vi "GV_PlotRscale.vi"(8 "error in (no error)":errorcluster, 11 "Gviewer in":refnum<class "Gviewer.lvclass">) -> (0 "error out":errorcluster, 3 "Gviewer out":refnum<class "Gviewer.lvclass">)   [LabVIEW 2020, in "Sgraph_lib_V1.lvlib" / "Gviewer.lvclass"]
doc: "Andre Koelewijn, 17 feb 2022,\n\nPlot Right Scale data if selected"
uses:
  Gviewer.lvclass
  Gviewer.lvclass/Gviewer.ctl
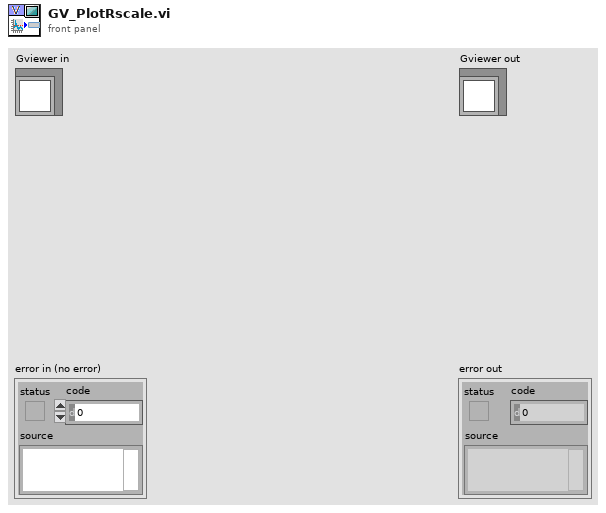
[diagram p1: front panel]
types:
  T1 = typedef "Sgraph_lib_V1.lvlib/Gviewer.lvclass/TD_Rscale.ctl" = enum16{"none", "one", "all"}
  T2 = typedef "Sgraph_lib_V1.lvlib/Gviewer.lvclass/Typedef_SelProperties.ctl" = cluster{"Color":u32, "LineType":T3, "max":dbl, "min":dbl, "unit":string}
  T3 = typedef "Sgraph_lib_V1.lvlib/Gviewer.lvclass/Typedef_LineType.ctl" = enum16{"num_bare", "num_MinMax_Area", "num_MinMax_Lines", "num_MinMax_Forfor", "num_Max_Area", "num_Max_Line", "num_Max_Forfor", "num_Min_Area", "num_Min_Line", "num_Min_Fosfor", "Boolean_Line_01", "Boolean_Area_01", "Boolean_Fosfor_01", "Boolean_Line_TF", "Boolean_Area_TF", "Boolean_Fosfor_TF", "Boolean_OnOff_Line", "Boolean_OnOff_Area", "Boolean_OnOff_Fosfor", "Boolean_spare", "StringEvent_Line", "StringEvent_TimeLine"}
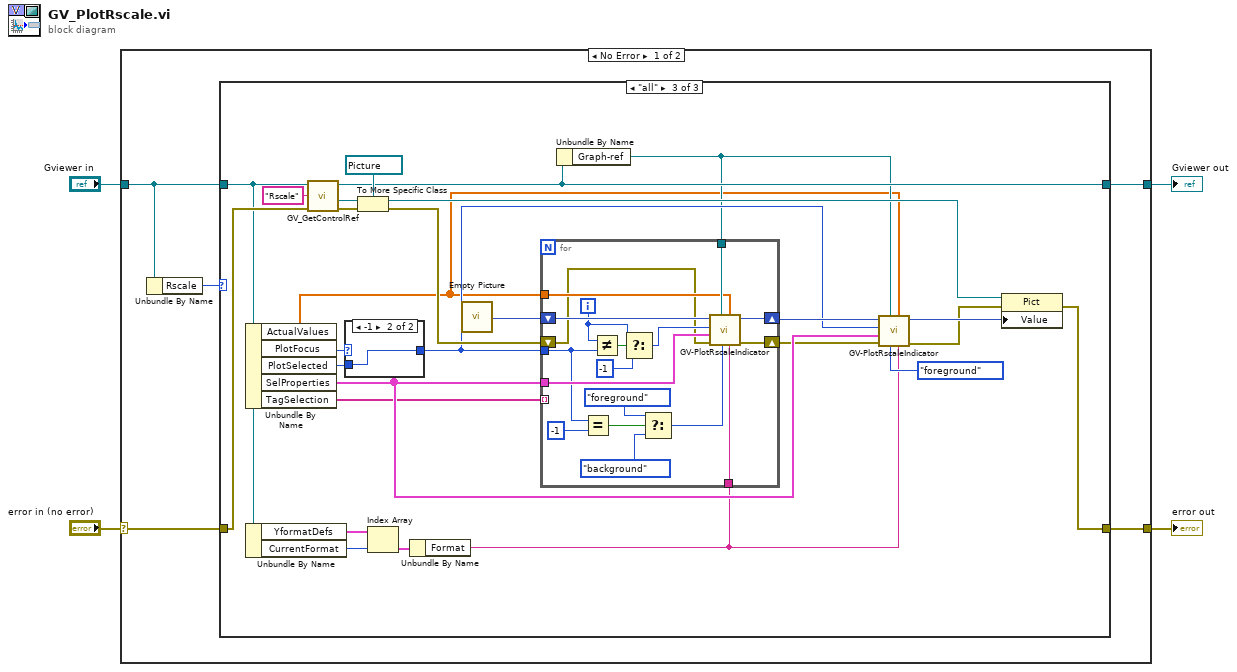
[diagram p0: block diagram]
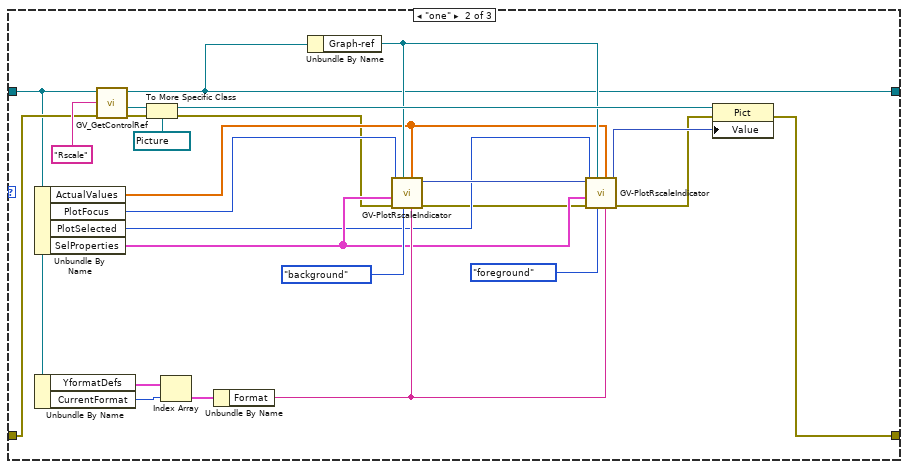
[diagram p3: hidden frame]
diagram:
  n1 = case shown="No Error" "error in (no error)" {
    selector: "error in (no error)" -> [w6 w85]
    tunnel: [w5 w85] -> w3
    tunnel: [w7 w84] -> w1
    tunnel: "Gviewer in" -> [w8 w84]
    frame No Error {
      n2 = Unbundle By Name(w8) -> ("Rscale"=w9:T1)
      n3 = case shown="\"all\"" w9 {
        tunnel: w8 -> [w11 w24 w55]
        tunnel: [w11 w12 w57] -> w7
        tunnel: w6 -> [w10 w31 w58]
        tunnel: [w10 w36 w63] -> w5
        frame Default {
        }
        frame "one" {
          n4 = Unbundle By Name(w24) -> ("ActualValues"=w17:dbl[], "PlotFocus"=w16:i32, "PlotSelected"=w15:i32, "SelProperties"=w18:T2[])
          n5 = Unbundle By Name(w24) -> ("YformatDefs"=w27:cluster{"Description":string, "Format":string}[], "CurrentFormat"=w26:i32)
          n6 = call "GV_GetControlRef.vi"("error in (no error)"=w31, "CNT name"="Rscale", "Gviewer in"=w24) -> ("error out"=w35:errorcluster, "Reference"=w34:refnum<vi>, "Gviewer out"=w12:refnum<class "Gviewer.lvclass">)  [unwired: 6 in]
          n7 = To More Specific Class(target class=refnum<vi> refnum ("2D Picture"), reference=w34, error in=w35) -> (specific class reference=w28:refnum<vi>, error out=w14:errorcluster)
          n8 = Index Array(array=w27, index=w26) -> (element=w25:cluster{"Description":string, "Format":string})
          n9 = Unbundle By Name(w25) -> ("Format"=w20:string)
          n10 = Unbundle By Name(w12) -> ("Graph-ref"=w21:refnum<vi>)
          n11 = call "GV-PlotRscaleIndicator.vi"("Format"=w20, "ActualValues"=w17, "type"=enum16{"background", "foreground"}."background", "Graph-ref"=w21, "error in (no error)"=w14, "SelProperties"=w18, "Plot"=w16) -> ("error out"=w13:errorcluster, "Picture OUT"=w23:picture)  [unwired: 3 in]
          n12 = call "GV-PlotRscaleIndicator.vi"("Format"=w20, "ActualValues"=w17, "type"=enum16{"background", "foreground"}."foreground", "Graph-ref"=w21, "error in (no error)"=w13, "SelProperties"=w18, "Plot"=w15, "Picture IN"=w23) -> ("error out"=w29:errorcluster, "Picture OUT"=w30:picture)  [unwired: 2 in]
          n13 = property class="Pict"(reference=w28, error in=w29, "Value"=w30) -> (error out=w36:errorcluster)  [unwired: 1 out]
        }
        frame "all" {
          n14 = Unbundle By Name(w55) -> ("ActualValues"=w37:dbl[], "PlotFocus"=w52:i32, "PlotSelected"=w51:i32, "SelProperties"=w46:T2[], "TagSelection"=w38:string[])
          n15 = Unbundle By Name(w55) -> ("YformatDefs"=w42:cluster{"Description":string, "Format":string}[], "CurrentFormat"=w41:i32)
          n16 = call "GV_GetControlRef.vi"("error in (no error)"=w58, "CNT name"="Rscale", "Gviewer in"=w55) -> ("error out"=w62:errorcluster, "Reference"=w61:refnum<vi>, "Gviewer out"=w57:refnum<class "Gviewer.lvclass">)  [unwired: 6 in]
          n17 = case shown="-1" w52 {
            selector: w52 -> [w64 _]
            tunnel: [w64 w65] -> w49
            tunnel: w51 -> [_ w65]
            frame Default {
            }
            frame -1 {
            }
          }
          n18 = To More Specific Class(target class=refnum<vi> refnum ("2D Picture"), reference=w61, error in=w62) -> (specific class reference=w56:refnum<vi>, error out=w53:errorcluster)
          n19 = Index Array(array=w42, index=w41) -> (element=w40:cluster{"Description":string, "Format":string})
          n20 = Unbundle By Name(w40) -> ("Format"=w39:string)
          n21 = call "Empty Picture"() -> ("empty picture"=w54:picture)
          n22 = Unbundle By Name(w57) -> ("Graph-ref"=w47:refnum<vi>)
          n23 = for {
            tunnel: w47 -> [w82]
            tunnel: w46 -> [w81]
            shift-right: [w83] -> w50
            shift-left: w54 -> [w80]
            shift-right: [w79] -> w45
            shift-left: w53 -> [w66]
            tunnel: w49 -> [w73]
            tunnel: w39 -> [w75]
            tunnel: w38 -> [_] mode=indexing
            tunnel: w37 -> [w68]
            i -> [w77]
            n24 = Equal?(x=w73, y=-1 ("f")) -> (x = y?=w72:bool)
            n25 = Not Equal?(x=w77, y=w73) -> (x != y?=w78:bool)
            n26 = Select(t=w77, s=w78, f=-1) -> (s? t:f=w67:i32)
            n27 = Select(t=enum16{"background", "foreground"}."foreground" ("type"), s=w72, f=enum16{"background", "foreground"}."background" ("type")) -> (s? t:f=w69:enum16{"background", "foreground"})
            n28 = call "GV-PlotRscaleIndicator.vi"("Format"=w75, "ActualValues"=w68, "type"=w69, "Graph-ref"=w82, "error in (no error)"=w66, "SelProperties"=w81, "Plot"=w67, "Picture IN"=w80) -> ("error out"=w79:errorcluster, "Picture OUT"=w83:picture)  [unwired: 2 in]
          }
          n29 = call "GV-PlotRscaleIndicator.vi"("Format"=w39, "ActualValues"=w37, "type"=enum16{"background", "foreground"}."foreground", "Graph-ref"=w47, "error in (no error)"=w45, "SelProperties"=w46, "Plot"=w49, "Picture IN"=w50) -> ("error out"=w43:errorcluster, "Picture OUT"=w44:picture)  [unwired: 2 in]
          n30 = property class="Pict"(reference=w56, error in=w43, "Value"=w44) -> (error out=w63:errorcluster)  [unwired: 1 out]
        }
      }
    }
    frame Error {
    }
  }
  "error out" <- w3
  "Gviewer out" <- w1
